vi "DSF.Engine.Hardware Info.CPU.Set Caches.vi"(8 "error in (no error)":errorcluster, 10 "Caches":T1(array[cluster]), 11 "CPU Info in":refnum<class "DSF.Engine.Hardware Info.CPU.lvclass">) -> (0 "error out":errorcluster, 3 "CPU Info out":refnum<class "DSF.Engine.Hardware Info.CPU.lvclass">)   [LabVIEW 2017, in "DSF.Engine.lvlib" / "DSF.Engine.Hardware Info.CPU.lvclass"]
uses:
  DSF.Engine.Hardware Info.CPU.lvclass
  DSF.Engine.Hardware Info.CPU.lvclass/DSF.Engine.Hardware Info.CPU.ctl
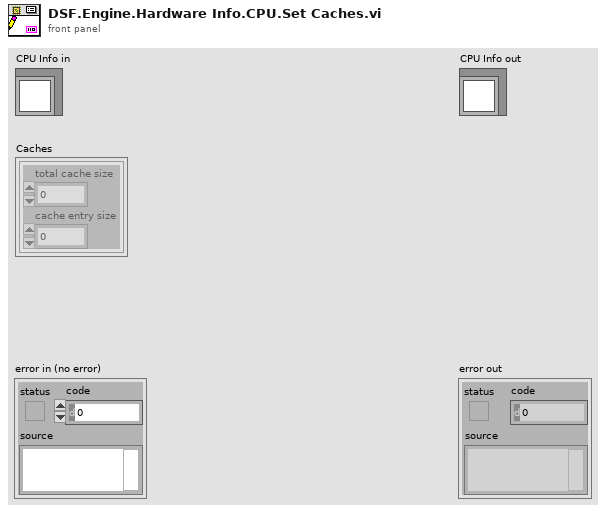
[diagram p1: front panel]
types:
  T1 = cluster{"total cache size":i32, "cache entry size":i32}[]
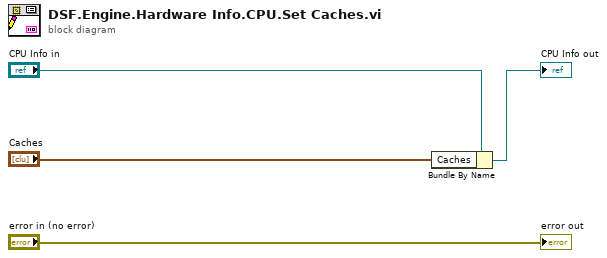
[diagram p0: block diagram]
diagram:
  n1 = Bundle By Name(cluster="CPU Info in", "Caches"="Caches") -> (→"CPU Info out":refnum<class "DSF.Engine.Hardware Info.CPU.lvclass">)
  "error out" <- "error in (no error)"
